vi "SubPanel Guest-Core_Initialize.vi"(0 "Initialization Sequence":string, 5 "FTW Actor Instance Configuration":string, 11 "error in (no error)":errorcluster) -> (4 "Actor Template-Core out":refnum<class "SubPanel Guest-Core.lvclass">, 6 "Incoming Requests":refnum<event-registration>, 8 "Local Messages":refnum<event-registration>, 15 "error out":errorcluster)   [LabVIEW 2018, in "SubPanel Guest-Core.lvclass"]
uses:
  SubPanel Guest-Core.lvclass
  source/CodeGen/JSON Deserialize/FTW-JSON-Deserialize.xnode
  source/CodeGen/JSON Deserialize/FTW-JSON-Core-GetFlattenedValue.vi
  source/Reflection/FTW-Reflection-Type.vi
  source/JSON/core/FTW-JSON-Core-EncodingFlags.vi
  source/JSON/FTW-JSON-Parse.vi
  source/actor/Message/Request/FTW-Message-IncomingRequest.lvclass
  C:/Jobs/Featherweight/featherweight-2018/source/actor/Message/Base/FTW-Message.lvclass
  source/actor/Message/Base/FTW-Message.lvclass
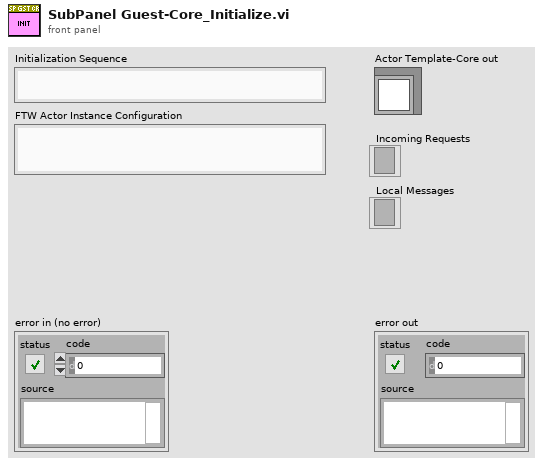
[diagram p1: front panel]
types:
  T1 = cluster{"Incoming Requests":refnum<event-registration>, "Local Messages":refnum<event-registration>, "Subscriber Registration":refnum<event-registration>}
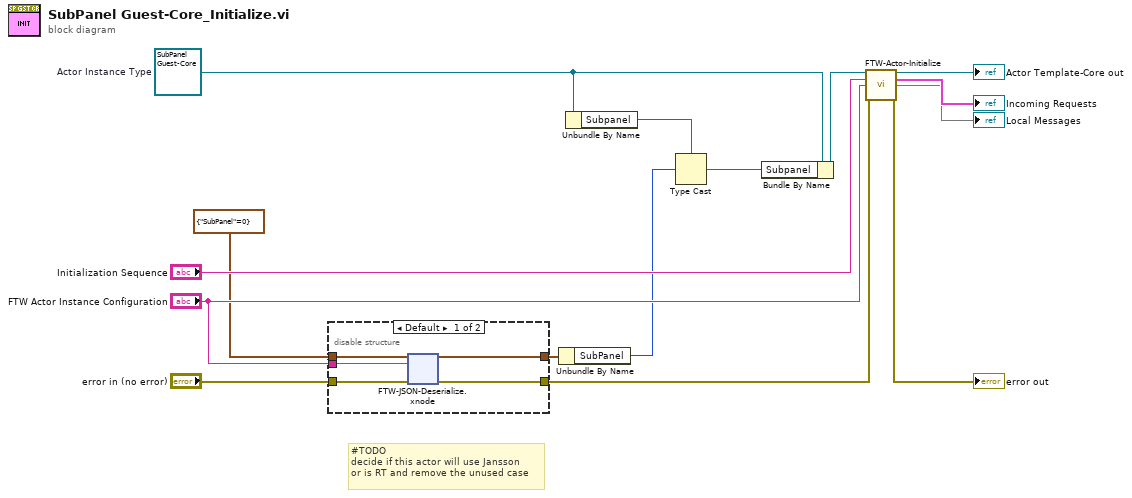
[diagram p0: block diagram]
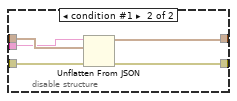
[diagram p2: hidden frame]
diagram:
  w4 = refnum<class "SubPanel Guest-Core.lvclass"> refnum  # Actor Instance Type
  # "#TODO\ndecide if this actor will use Jansson\nor is RT and remove the unused case"
  n1 = disable-structure shown="Default" {
    disable-tunnel: "error in (no error)" -> [w20 w37]
    disable-tunnel: [w19 w36] -> w10
    disable-tunnel: "FTW Actor Instance Configuration" -> [w18 w34]
    disable-tunnel: cluster{"SubPanel":i32} {"SubPanel"=0} ("Type and Defaults") -> [w17 w35]
    disable-tunnel: [w16 w33] -> w6
    frame condition #0 (active) {
      n2 = xnode "FTW-JSON-Deserialize.xnode"("Type and Defaults"=w17, "JSON String"=w18, "error in"=w20) -> ("Values"=w16:cluster{"SubPanel":i32}, "error out"=w19:errorcluster)
    }
    frame condition #1 {
      n3 = Unflatten From JSON(JSON string=w34, type and defaults=w35, error in (no error)=w37) -> (value=w33:cluster{"SubPanel":i32}, error out=w36:errorcluster)  [unwired: 4 in]
    }
  }
  n4 = Unbundle By Name(w6) -> ("SubPanel"=w2:i32)
  n5 = Unbundle By Name(w4) -> ("Subpanel"=w3:refnum<vi>)
  n6 = Type Cast(type=w3, x=w2) -> (*(type *) &x=w1:refnum<vi>)
  n7 = Bundle By Name(cluster=w4, "Subpanel"=w1) -> (w7:refnum<class "SubPanel Guest-Core.lvclass">)
  n8 = call-dynamic "FTW-Actor-Initialize.vi"("FTW Actor Instance Type"=w7, "Initialization Job Sequence"="Initialization Sequence", "Actor Instance Configuration"="FTW Actor Instance Configuration", "error in"=w10) -> ("FTW Actor Instance"=→"Actor Template-Core out":refnum<class "SubPanel Guest-Core.lvclass">, "Event Refnums"=→"Incoming Requests":T1, 8:→"Local Messages", "error out"=→"error out":errorcluster)  [unwired: 8 in]
